vi "数据查询.vi"() -> ()   [LabVIEW 2016, in "数据查询.lvlib"]
uses:
  <vilib>/Utility/sysdir.llb/System Directory Type.ctl
  <vilib>/Utility/miscctls.llb/LVPointTypeDef.ctl
  var/holding var.vi
  <vilib>/ptbypt/NI_PtbyPt.lvlib
panel:
  out "布尔":bool
  in  "设置按钮":bool
  in  "标识说明":bool
  in  "数据查询菜单":T1
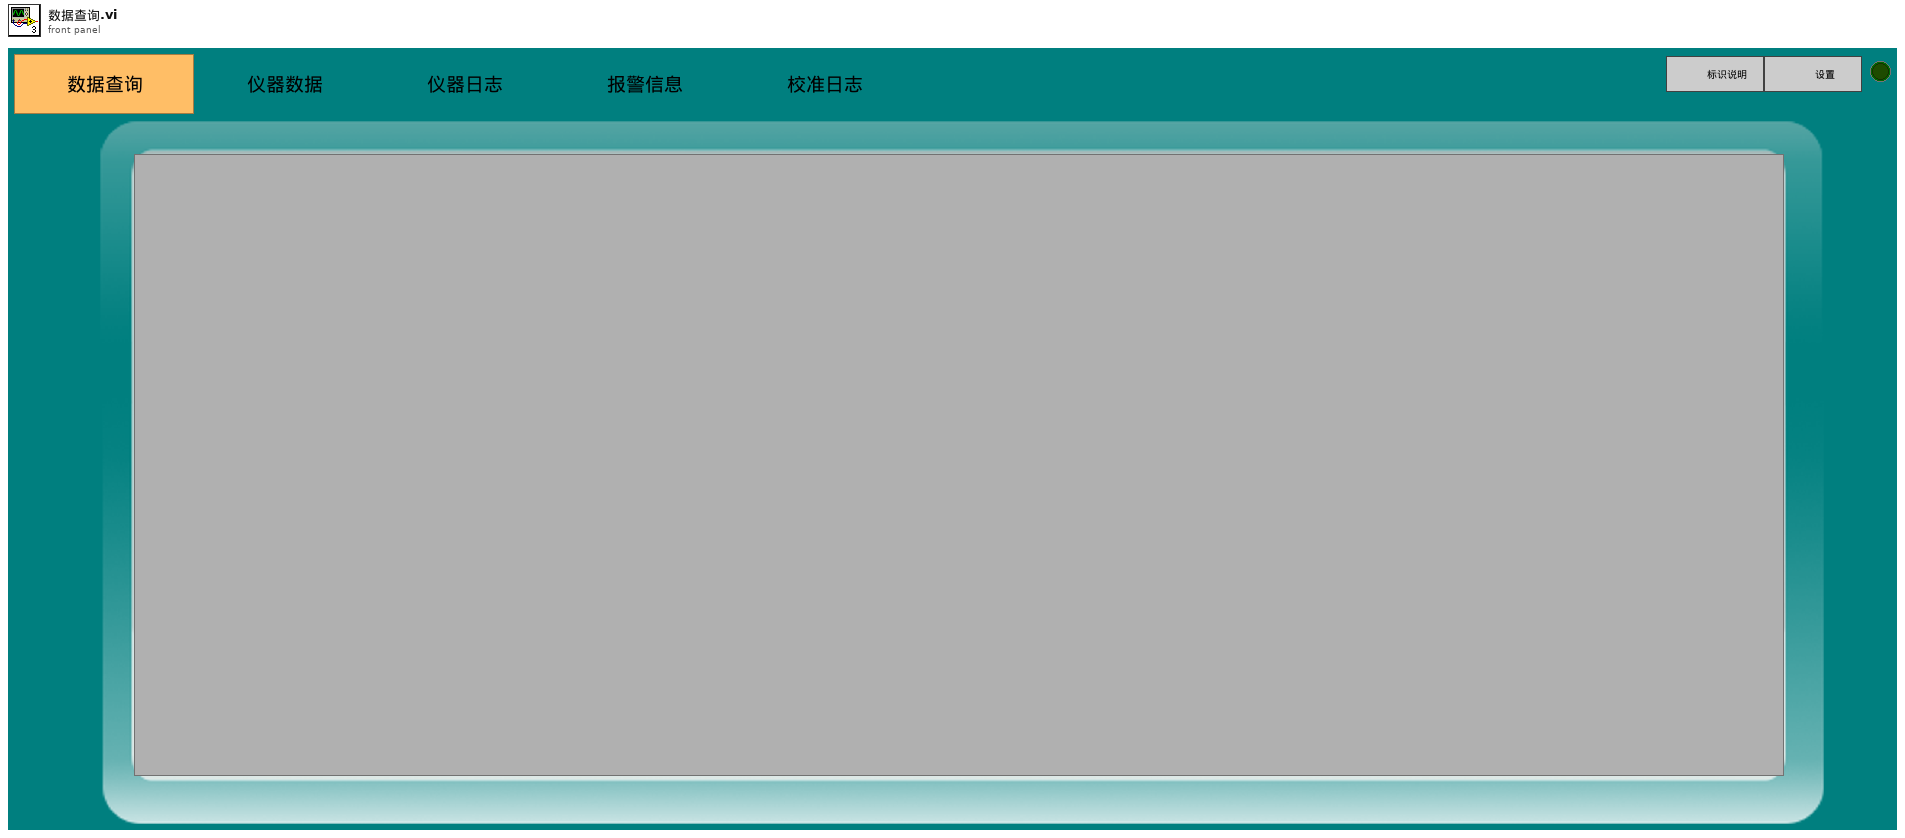
[diagram p1: front panel]
types:
  T1 = typedef "数据查询.lvlib/数据查询单选控件.ctl" = enum32{"数据查询", "仪器数据", "仪器日志", "报警信息", "校准日志"}
  T2 = typedef "LVPointTypeDef.ctl" = cluster{"Horizontal":i16, "Vertical":i16}
  T3 = typedef "System Directory Type.ctl" = i32
  T4 = typedef "LVDateTimeRec.ctl" = cluster{"秒数的小数部分":dbl, "秒":i32, "分":i32, "时":i32, "日":i32, "月":i32, "年":i32, "天数（周）":i32, "天数（年）":i32, "DST":i32}
  T5 = enum32{"Bad", "Idle", "Run top level", "Running"}
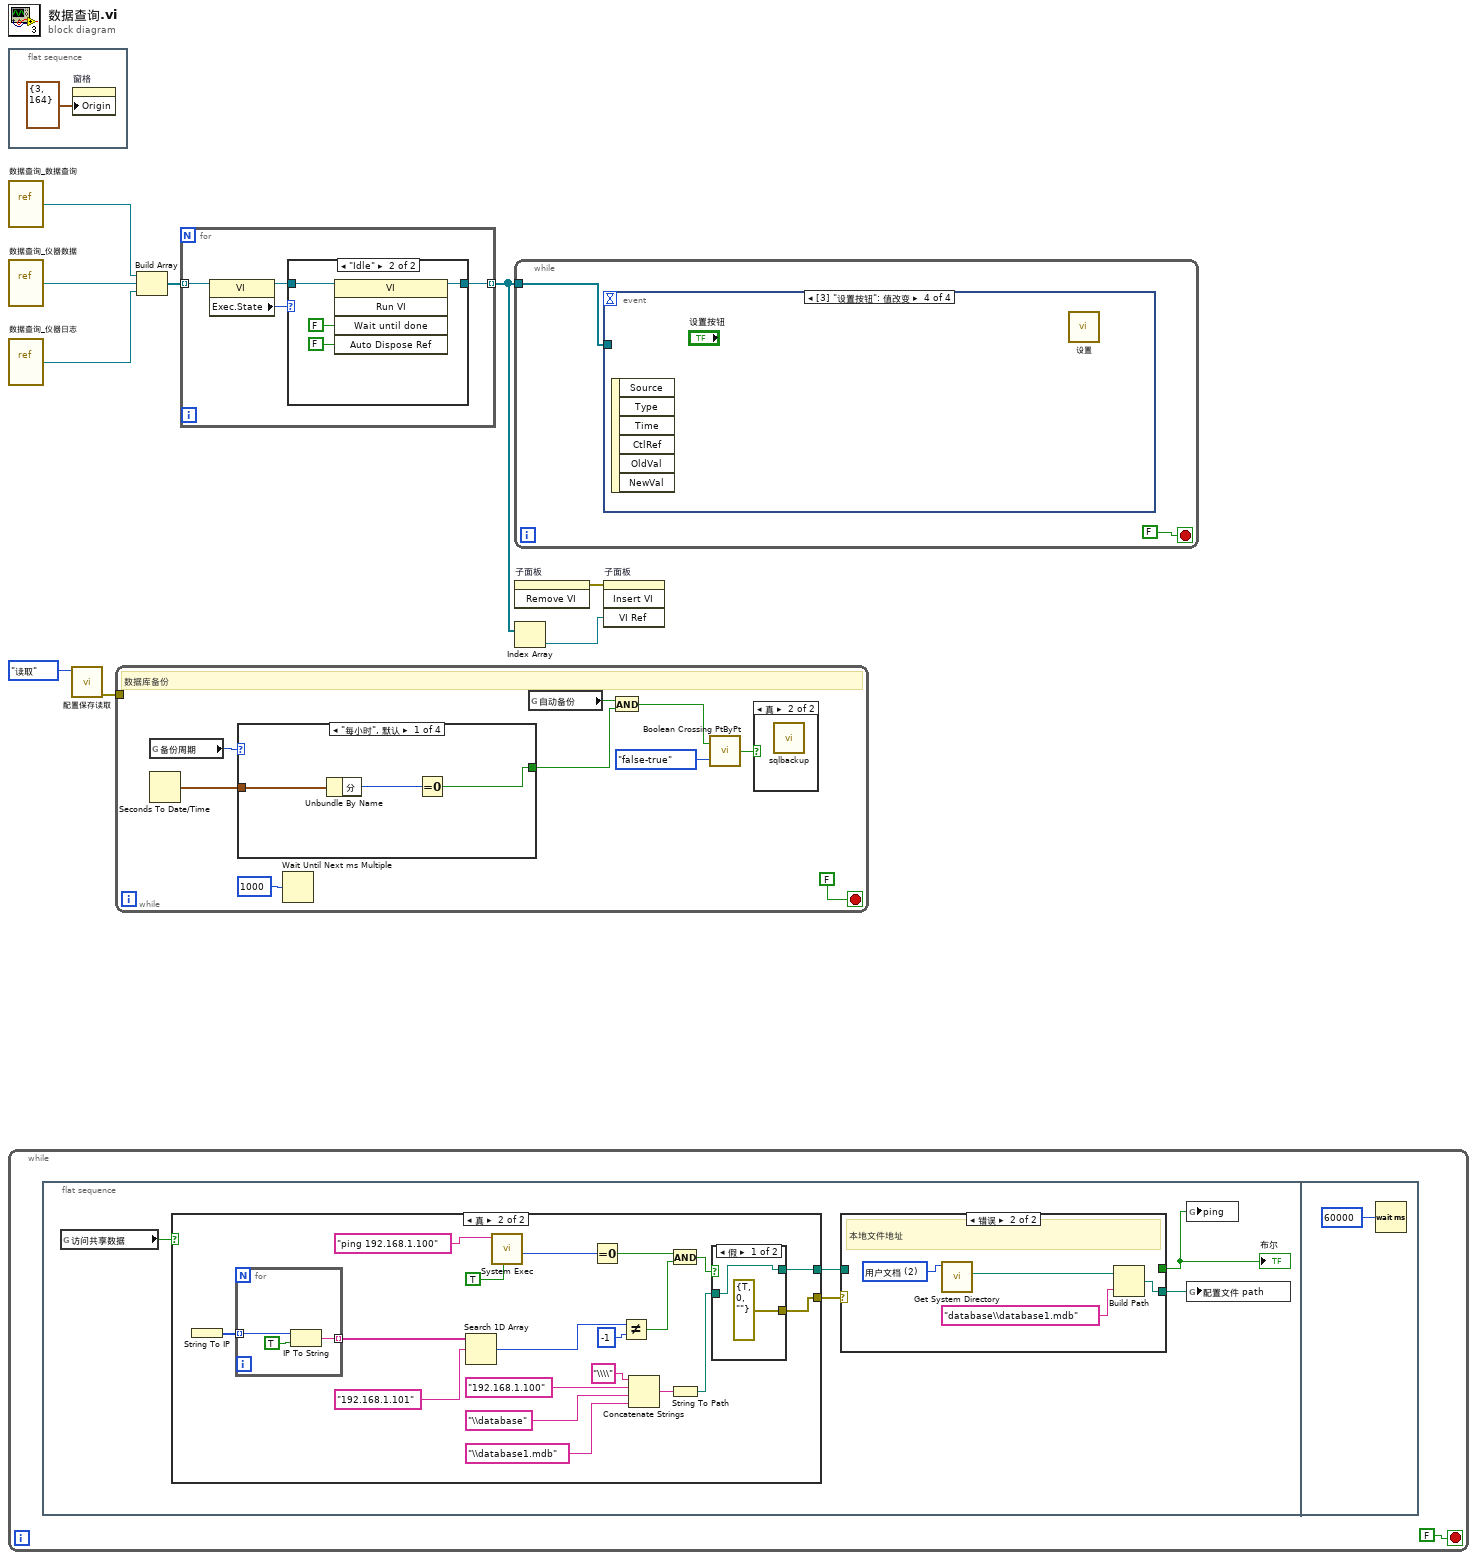
[diagram p0: block diagram]
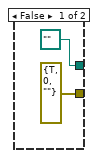
[diagram p2: hidden frame]
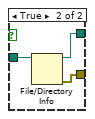
[diagram p3: hidden frame]
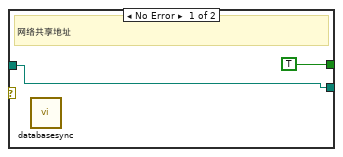
[diagram p4: hidden frame]
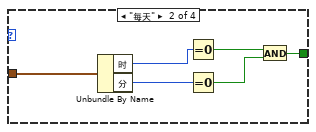
[diagram p6: hidden frame]
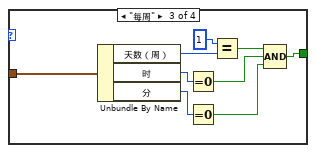
[diagram p7: hidden frame]
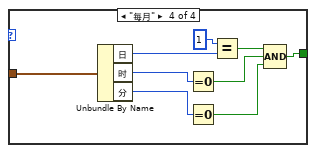
[diagram p8: hidden frame]
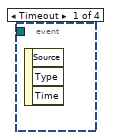
[diagram p10: hidden frame]
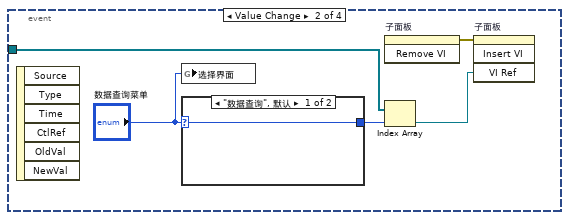
[diagram p11: hidden frame]
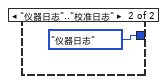
[diagram p12: hidden frame]
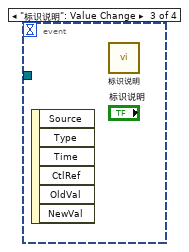
[diagram p13: hidden frame]
diagram:
  n1 = flat-sequence {
    frame #0 {
      n2 = property on="窗格" class="Pane"("Origin"=T2 {"Horizontal"=3, "Vertical"=164} ("原点")) -> ()  [unwired: 2 in, 2 out]
    }
  }
  n3 = vi-ref "数据查询_数据查询.vi"() -> (w6:refnum<vi>)
  n4 = vi-ref "数据查询_仪器数据.vi"() -> (w4:refnum<vi>)
  n5 = vi-ref "数据查询_仪器日志.vi"() -> (w3:refnum<vi>)
  n6 = while {
    stop <- FALSE stop-if-true
    n7 = flat-sequence {
      frame #0 {
        n8 = global read "全局变量.vi" "访问共享数据"() -> (w13:bool)
        n9 = case shown="真" w13 {
          tunnel: [path "" ("dup path") w31] -> w16
          tunnel: [errorcluster {"status"=TRUE, "code"=0, "source"=""} ("error out") w30] -> w15
          frame False {
          }
          frame True {
            n10 = String To IP() -> (0:w24:u32[])  [unwired: 1 in]
            n11 = for {
              tunnel: w24 -> [w40] mode=indexing
              tunnel: [w39] -> w23 mode=indexing
              n12 = IP To String(1:TRUE ("句点符号？(F)"), 2:w40) -> (0:w39:string)
            }
            n13 = Search 1D Array(1D array=w23, element="192.168.1.101" ("command line")) -> (index of element=w21:i32)  [unwired: 1 in]
            n14 = call <vilib>:"System Exec.vi"("run minimized? (F)"=TRUE, "command line"="ping 192.168.1.100") -> ("return code"=w27:i32)  [unwired: 6 in, 3 out]
            n15 = Equal To 0?(x=w27) -> (x = 0?=w26:bool)
            n16 = Not Equal?(x=w21, y=-1) -> (x != y?=w19:bool)
            n17 = Concatenate Strings("\\\\" ("字符串"), "192.168.1.100" ("名称"), "\\database" ("字符串"), "\\database1.mdb" ("名称或相对路径")) -> (w36:string)
            n18 = And(x=w26, y=w19) -> (x .and. y?=w25:bool)
            n19 = String To Path(string=w36) -> (path=w33:path)
            n20 = case shown="假" w25 {
              tunnel: w33 -> [w42 w45]
              tunnel: [w42 w44] -> w31
              tunnel: [errorcluster {"status"=TRUE, "code"=0, "source"=""} ("error out") w43] -> w30
              frame False {
              }
              frame True {
                n21 = File/Directory Info(path=w45) -> (path out=w44:path, error out=w43:errorcluster)  [unwired: 1 in, 5 out]
              }
            }
          }
        }
        n22 = case shown="错误" w15 {
          tunnel: w16 -> [w47 _]
          tunnel: [w47 w50] -> w14
          tunnel: [TRUE _] -> w12
          frame No Error {
            # "网络共享地址"
            n23 = call "databasesync.vi"() -> ()  [unwired: 12 in]
          }
          frame Error {
            w48 = T3 2 items=["用户目录"=0, "用户桌面"=1, "用户文档"=2, "用户应用程序数据"=3, "用户设置"=4, "用户临时目录"=5, "公共文档"=6, "公共应用程序数据"=7, "公共设置"=8, "公共缓存"=13, "系统核心库"=9, "系统安装库"=10, "应用程序文件"=11, "启动盘根目录"=12] ("system directory type")
            # "本地文件地址"
            n24 = call <vilib>:"Get System Directory.vi"("system directory type"=w48) -> ("system directory"=w49:path)  [unwired: 10 in]
            n25 = Build Path(base path=w49, name or relative path="database\\database1.mdb" ("名称或相对路径")) -> (appended path=w50:path)
          }
        }
        "布尔" <- w12
        n26 = global write "全局变量.vi" "ping"(w12) -> ()
        n27 = global write "全局变量.vi" "配置文件 path"(w14) -> ()
      }
      frame #1 {
        n28 = Wait (ms)(milliseconds to wait=u32 60000 ("等待时间（毫秒）")) -> ()  [unwired: 1 out]
      }
    }
  }
  n29 = call "配置保存读取.vi"("配置"=enum16{"读取", "写入"}."读取") -> ("error out"=w1:errorcluster)  [unwired: 10 in]
  n30 = while {
    tunnel: w1 -> [_]
    stop <- FALSE stop-if-true
    # "数据库备份"
    n31 = global read "holding var.vi" "备份周期"() -> (w60:enum16{"每小时", "每天", "每周", "每月"})
    n32 = Seconds To Date/Time() -> (date time rec=w55:T4)  [unwired: 2 in]
    n33 = case shown="\"每小时\", 默认" w60 {
      tunnel: w55 -> [w64 w70 w79 w88]
      tunnel: [w62 w65 w71 w80] -> w54
      frame "每小时", Default {
        n34 = Unbundle By Name(w64) -> ("分"=w63:i32)
        n35 = Equal To 0?(x=w63) -> (x = 0?=w62:bool)
      }
      frame "每天" {
        n36 = Unbundle By Name(w70) -> ("时"=w68:i32, "分"=w69:i32)
        n37 = Equal To 0?(x=w68) -> (x = 0?=w66:bool)
        n38 = Equal To 0?(x=w69) -> (x = 0?=w67:bool)
        n39 = And(x=w66, y=w67) -> (x .and. y?=w65:bool)
      }
      frame "每周" {
        n40 = Unbundle By Name(w79) -> ("天数（周）"=w78:i32, "时"=w76:i32, "分"=w75:i32)
        n41 = Equal To 0?(x=w76) -> (x = 0?=w73:bool)
        n42 = Equal To 0?(x=w75) -> (x = 0?=w72:bool)
        n43 = Equal?(x=1, y=w78) -> (x = y?=w74:bool)
        n44 = Compound Arithmetic op=AND ("复合运算")(w74, w73, w72) -> (w71:bool)
      }
      frame "每月" {
        n45 = Unbundle By Name(w88) -> ("日"=w87:i32, "时"=w85:i32, "分"=w84:i32)
        n46 = Equal To 0?(x=w85) -> (x = 0?=w82:bool)
        n47 = Equal To 0?(x=w84) -> (x = 0?=w81:bool)
        n48 = Equal?(x=1, y=w87) -> (x = y?=w83:bool)
        n49 = Compound Arithmetic op=AND ("复合运算")(w83, w82, w81) -> (w80:bool)
      }
    }
    n50 = Wait Until Next ms Multiple(millisecond multiple=u32 1000 ("毫秒倍数")) -> ()  [unwired: 1 out]
    n51 = global read "holding var.vi" "自动备份"() -> (w59:bool)
    n52 = And(x=w59, y=w54) -> (x .and. y?=w58:bool)
    n53 = call <vilib>:"Boolean Crossing PtByPt.vi"("direction"=enum16{"either", "false-true", "true-false"}."false-true", "input"=w58) -> ("crossing"=w56:bool)  [unwired: 1 in]
    n54 = case shown="真" w56 {
      frame False {
      }
      frame True {
        n55 = call "sqlbackup.vi"() -> ()  [unwired: 11 in, 1 out]
      }
    }
  }
  n56 = Build Array(w6, w4, w3) -> (w5:refnum<vi>[])
  n57 = for {
    tunnel: w5 -> [w92] mode=indexing
    tunnel: [w89] -> w8 mode=indexing
    n58 = property class="VI"(reference=w92) -> (reference out=w90:refnum<vi>, "Exec.State"=w91:T5)  [unwired: 1 in, 1 out]
    n59 = case shown="\"Idle\"" w91 {
      tunnel: w90 -> [w93 w95]
      tunnel: [w93 w94] -> w89
      frame "Bad", Default {
      }
      frame "Idle" {
        n60 = invoke class="VI" method="Run VI"(reference=w95, "Wait until done"=FALSE ("结束前等待"), "Auto Dispose Ref"=FALSE ("自动销毁引用")) -> (reference out=w94:refnum<vi>)  [unwired: 2 in, 4 out]
      }
    }
  }
  n61 = while {
    tunnel: w8 -> [w98]
    stop <- FALSE stop-if-true
    n62 = event shown="[3] \"设置按钮\": 值改变" {
      selector: _ -> [_ _ _ _]
      dyn-events: _ -> [_ _ _ _]
      timeout: _ -> [_ _ _ _]
      tunnel: w98 -> [_ w104 _ _]
      event Timeout {
        n63 = event-data() -> ()  [unwired: 1 in, 3 out]
      }
      event Value Change {
        n64 = event-data() -> ()  [unwired: 1 in, 6 out]
        n65 = global write "全局变量.vi" "选择界面"("数据查询菜单") -> ()
        n66 = case shown="\"数据查询\", 默认" "数据查询菜单" {
          selector: "数据查询菜单" -> [w105 _]
          tunnel: [w105 enum32{"数据查询", "仪器数据", "仪器日志", "报警信息", "校准日志"}."仪器日志" ("数据查询菜单")] -> w101
          frame "数据查询", Default {
          }
          frame "仪器日志".."校准日志" {
          }
        }
        n67 = invoke on="子面板" class="SubPnl" method="Remove VI"() -> (error out=w102:errorcluster)  [unwired: 3 in, 2 out]
        n68 = Index Array(array=w104, index=w101) -> (element=w103:refnum<vi>)
        n69 = invoke on="子面板" class="SubPnl" method="Insert VI"(error in=w102, "VI Ref"=w103) -> ()  [unwired: 2 in, 4 out]
      }
      event "标识说明": Value Change {
        n70 = event-data() -> ()  [unwired: 1 in, 6 out]
        n71 = call "标识说明.vi"() -> ()  [unwired: 12 in]
      }
      event "设置按钮": Value Change {
        n72 = event-data() -> ()  [unwired: 1 in, 6 out]
        n73 = call "设置.vi"() -> ()  [unwired: 12 in]
      }
    }
  }
  n74 = invoke on="子面板" class="SubPnl" method="Remove VI"() -> (error out=w9:errorcluster)  [unwired: 3 in, 2 out]
  n75 = Index Array(array=w8) -> (element=w7:refnum<vi>)  [unwired: 1 in]
  n76 = invoke on="子面板" class="SubPnl" method="Insert VI"(error in=w9, "VI Ref"=w7) -> ()  [unwired: 2 in, 4 out]
